vi "Create.vi"(8 "error in (no error)":errorcluster, 11 "Option String (\"\")":string) -> (0 "error out":errorcluster, 3 "Session Factory out":refnum<class "Session Factory.lvclass">)   [LabVIEW 2021, in "NI Session Management niSE.lvlib" / "Session Factory.lvclass"]
uses:
  Session Factory.lvclass
  Session Factory.lvclass/Session Factory.ctl
panel:
  in  "Session Factory in":refnum<class "Session Factory.lvclass">
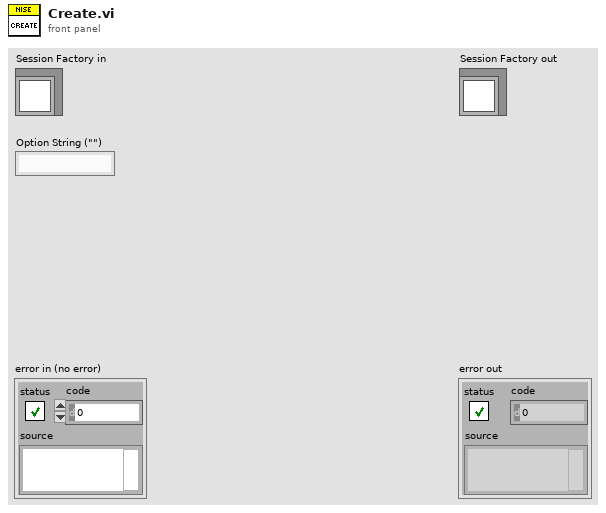
[diagram p1: front panel]
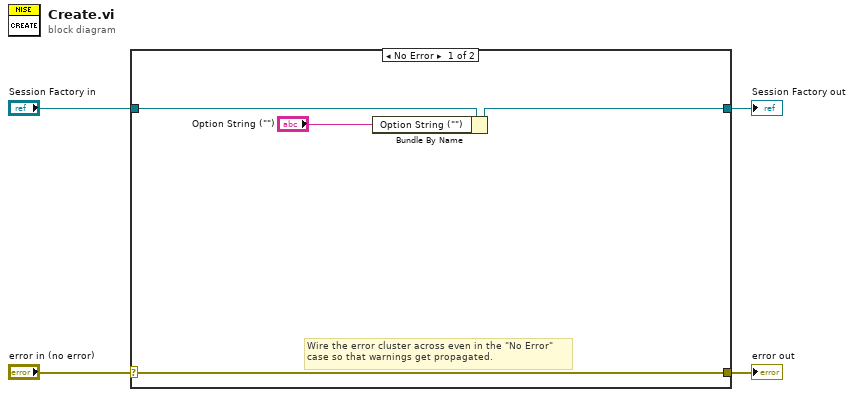
[diagram p0: block diagram]
diagram:
  n1 = case shown="No Error" "error in (no error)" {
    selector: "error in (no error)" -> [w7 w10]
    tunnel: [w7 w10] -> w3
    tunnel: [w6 w9] -> w1
    tunnel: "Session Factory in" -> [w8 w9]
    frame No Error {
      # "Wire the error cluster across even in the \"No Error\"\ncase so that warnings get propagated."
      n2 = Bundle By Name(cluster=w8, "Option String (\"\")"="Option String (\"\")") -> (w6:refnum<class "Session Factory.lvclass">)
    }
    frame Error {
    }
  }
  "error out" <- w3
  "Session Factory out" <- w1
